vi "Not structured type.vi"() -> (0 "error out":errorcluster)   [LabVIEW 2015]
uses:
  <vilib>/Utility/error.llb/DialogType.ctl
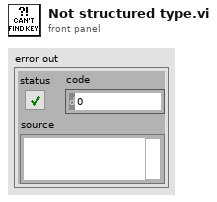
[diagram p1: front panel]
types:
  T1 = typedef "DialogType.ctl" = u16
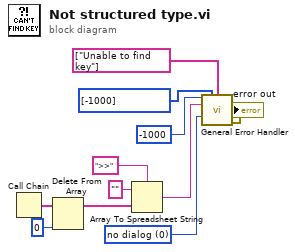
[diagram p0: block diagram]
diagram:
  w9 = T1 0 items=["no dialog", "OK message", "continue or stop message", "OK message + warnings", "continue/stop + warnings"] ("type of dialog (OK msg:1)")
  n1 = Call Chain() -> (call chain=w4:string[])
  n2 = Delete From Array(array=w4, index=0) -> (array with subset deleted=w6:string[])  [unwired: 1 in, 1 out]
  n3 = Array To Spreadsheet String(delimiter (Tab)=">>", array=w6, 3:"" ("format string")) -> (spreadsheet string=w5:string)
  n4 = call <vilib>:"General Error Handler.vi"("[error code] (0)"=-1000 ("error code (no error:0)"), "[user-defined codes]"=i32[] [-1000], "[user-defined descriptions]"=string[] ["Unable to find key"], "[error source] (\" \")"=w5, "type of dialog (OK msg:1)"=w9) -> ("error out"=→"error out":errorcluster)  [unwired: 6 in, 4 out]
